vi "CSTK_Icon Creator.vi"   [LabVIEW 2015]
uses:
  Library/Icon Creator/CSTK_Icon Creator.lvlib
panel:
  # "Icon Creator"
types:
  T1 = enum32{"Invalid", "Standard", "Closed", "Hidden", "Minimized", "Maximized"}
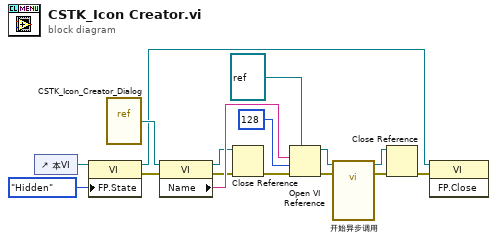
[diagram p0: block diagram]
diagram:
  n1 = control-ref of="本VI"() -> (w15:refnum<vi>)
  n2 = property class="VI"(reference=w15, "FP.State"=T1."Hidden" ("前面板窗口:状态")) -> (reference out=w6:refnum<vi>, error out=w5:errorcluster)  [unwired: 1 in]
  n3 = vi-ref "CSTK_Icon_Creator_Dialog.vi"() -> (w13:refnum<vi>)
  n4 = property class="VI"(reference=w13, error in=w5) -> (reference out=w3:refnum<vi>, error out=w2:errorcluster, "Name"=w16:string)
  n5 = Close Reference(reference=w3, error in (no error)=w2) -> (error out=w1:errorcluster)
  n6 = Open VI Reference(type specifier VI Refnum (for type only)=refnum<vi> refnum ("类型说明符VI引用句柄（仅用于类型）"), vi path=w16, options=128 ("选项"), error in (no error)=w1) -> (vi reference=w4:refnum<vi>, error out=w11:errorcluster)  [unwired: 2 in]
  n7 = call-by-ref "开始异步调用"(reference=w4, error in=w11) -> (reference out=w10:refnum<vi>, error out=w9:errorcluster)  [unwired: 12 in]
  n8 = Close Reference(reference=w10, error in (no error)=w9) -> (error out=w7:errorcluster)
  n9 = invoke class="VI" method="FP.Close"(reference=w6, error in=w7) -> ()  [unwired: 1 in, 3 out]
